vi "Columns.vi"() -> (2 "Columns":T1)   [LabVIEW 2020, in "Conditum-Tools.lvlib" / "NewEntityTemplate.lvclass"]
uses:
  NewEntityTemplate.lvclass
  NewEntityTemplate.lvclass/NewEntityTemplate.ctl
  Columns.ctl
  Conditum/Columns/Type/Type.lvclass
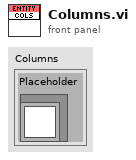
[diagram p1: front panel]
types:
  T1 = typedef "Conditum-Tools.lvlib/NewEntityTemplate.lvclass/Columns.ctl" = cluster{"Placeholder":refnum<class "Type.lvclass">}
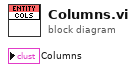
[diagram p0: block diagram]
diagram:
